vi "CAL_LOAD_R.vi"(9 "Control param In":T1={"L_velocity"=10000, "L_Power"=0.0, "R_velocity"=10000, "R_Power"=0.0, "T_param_L"={"Onset start"=0.0, "Onset end"=5.0, "Peak start"=10.0, "Release start"=60.0, "slang"=80.0, "Peak end"=58.0}, "T_param_R"={"Onset start"=0.0, "Onset end"=5.0, "Peak start"=10.0, "Release start"=60.0, "slang"=80.0, "Peak end"=58.0}, "Initialize?"=FALSE, "CAN read?"=FALSE, "Optimal count"=0}, 10 "Force":sgl[](array[numeric]), 11 "Param In":T2) -> (3 "Param Out":T2, 5 "Load_Peak":sgl, 7 "Load_Onset":sgl)   [LabVIEW 2019]
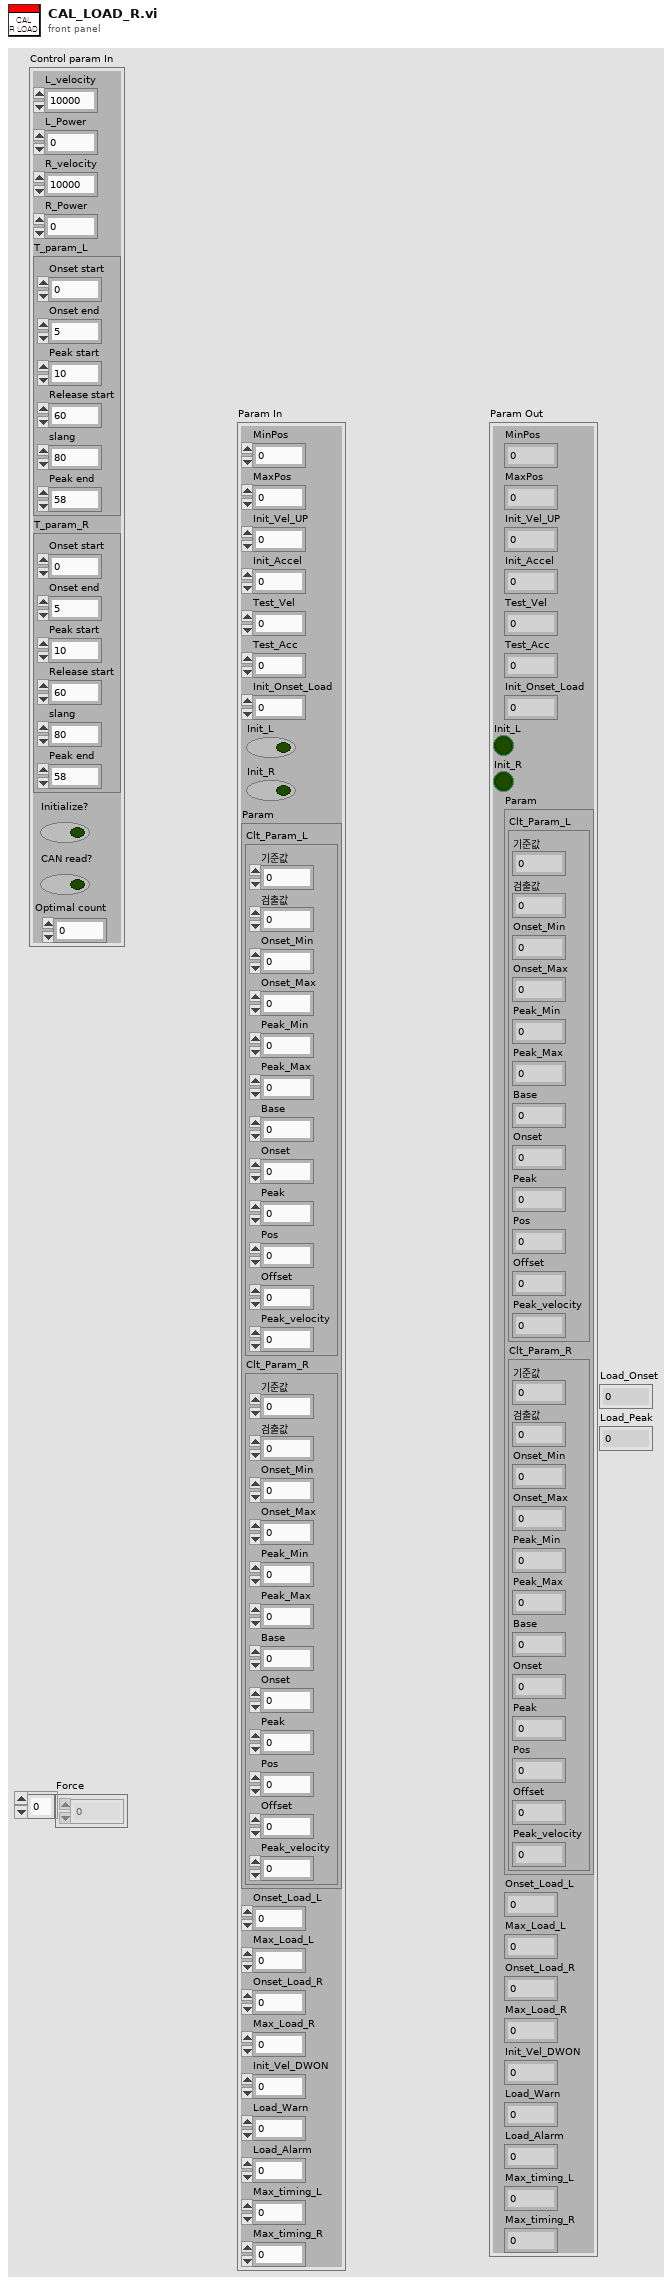
[diagram p1: front panel]
types:
  T1 = cluster{"L_velocity":u32, "L_Power":sgl, "R_velocity":u32, "R_Power":sgl, "T_param_L":cluster{"Onset start":sgl, "Onset end":sgl, "Peak start":sgl, "Release start":sgl, "slang":sgl, "Peak end":sgl}, "T_param_R":cluster{"Onset start":sgl, "Onset end":sgl, "Peak start":sgl, "Release start":sgl, "slang":sgl, "Peak end":sgl}, "Initialize?":bool, "CAN read?":bool, "Optimal count":i32}
  T2 = cluster{"MinPos":i32, "MaxPos":i32, "Init_Vel_UP":i32, "Init_Accel":u32, "Test_Vel":i32, "Test_Acc":u32, "Init_Onset_Load":sgl, "Init_L":bool, "Init_R":bool, "Param":cluster{"Clt_Param_L":cluster{"기준값":sgl, "검출값":sgl, "Onset_Min":sgl, "Onset_Max":sgl, "Peak_Min":sgl, "Peak_Max":sgl, "Base":i32, "Onset":i32, "Peak":i32, "Pos":i32, "Offset":sgl, "Peak_velocity":i32}, "Clt_Param_R":cluster{"기준값":sgl, "검출값":sgl, "Onset_Min":sgl, "Onset_Max":sgl, "Peak_Min":sgl, "Peak_Max":sgl, "Base":i32, "Onset":i32, "Peak":i32, "Pos":i32, "Offset":sgl, "Peak_velocity":i32}}, "Onset_Load_L":sgl, "Max_Load_L":sgl, "Onset_Load_R":sgl, "Max_Load_R":sgl, "Init_Vel_DWON":i32, "Load_Warn":sgl, "Load_Alarm":sgl, "Max_timing_L":sgl, "Max_timing_R":sgl}
  T3 = cluster{"Onset start":sgl, "Onset end":sgl, "Peak start":sgl, "Release start":sgl, "slang":sgl, "Peak end":sgl}
  T4 = cluster{"Onset start":i32, "Onset end":i32, "Peak start":i32, "Release start":i32, "slang":i32, "Peak end":i32}
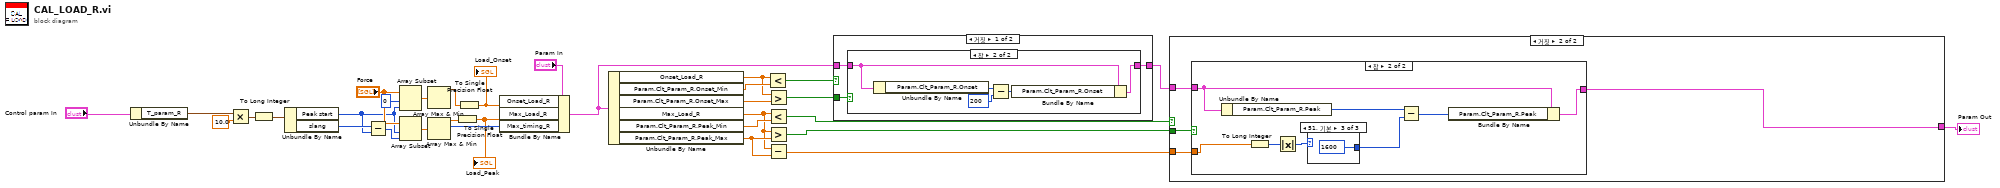
[diagram p0: block diagram]
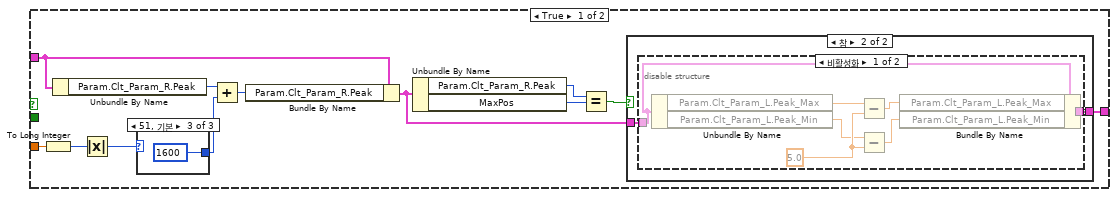
[diagram p2: hidden frame]
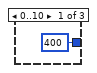
[diagram p5: hidden frame]
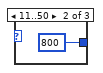
[diagram p6: hidden frame]
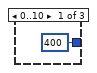
[diagram p8: hidden frame]
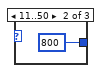
[diagram p9: hidden frame]
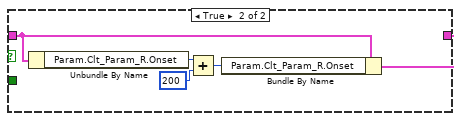
[diagram p11: hidden frame]
diagram:
  n1 = Unbundle By Name("Control param In") -> ("T_param_R"=w6:T3)
  n2 = Multiply(x=w6, y=sgl 10.0) -> (x*y=w22:T3)
  n3 = To Long Integer(number=w22) -> (32bit integer=w21:T4)
  n4 = Unbundle By Name(w21) -> ("Peak start"=w7:i32, "slang"=w14:i32)
  n5 = Subtract(x=w14, y=w7) -> (x-y=w8:i32)
  n6 = Array Subset(array="Force", index=0 ("인덱스"), length=w7) -> (w18:sgl[])
  n7 = Array Subset(array="Force", index=w7, length=w8) -> (w16:sgl[])
  n8 = Array Max & Min(array=w18) -> (max value=w10:sgl)  [unwired: 3 out]
  n9 = Array Max & Min(array=w16) -> (max value=w12:sgl, max index (indices)=w13:i32)  [unwired: 2 out]
  n10 = To Single Precision Float(number=w12) -> (single precision float=w11:sgl)
  "Load_Peak" <- w11
  n11 = To Single Precision Float(number=w10) -> (single precision float=w9:sgl)
  "Load_Onset" <- w9
  n12 = Bundle By Name(cluster="Param In", "Onset_Load_R"=w9, "Max_Load_R"=w11, "Max_timing_R"=w13) -> (w19:T2)
  n13 = Unbundle By Name(w19) -> ("Onset_Load_R"=w30:sgl, "Param.Clt_Param_R.Onset_Min"=w32:sgl, "Param.Clt_Param_R.Onset_Max"=w31:sgl, "Max_Load_R"=w2:sgl, "Param.Clt_Param_R.Peak_Min"=w29:sgl, "Param.Clt_Param_R.Peak_Max"=w3:sgl)
  n14 = Less?(x=w30, y=w32) -> (x < y?=w28:bool)
  n15 = Greater?(x=w30, y=w31) -> (0:w27:bool)
  n16 = Less?(x=w2, y=w29) -> (x < y?=w25:bool)
  n17 = Greater?(x=w2, y=w3) -> (0:w24:bool)
  n18 = Subtract(x=w2, y=w3) -> (x-y=w1:sgl)
  n19 = case shown="거짓" w28 {
    tunnel: w19 -> [w35 w43]
    tunnel: w27 -> [w33 _]
    tunnel: [w34 w42] -> w26
    frame False {
      n20 = case shown="참" w33 {
        tunnel: w35 -> [w36 w39]
        tunnel: [w36 w37] -> w34
        frame False {
        }
        frame True {
          n21 = Unbundle By Name(w39) -> ("Param.Clt_Param_R.Onset"=w41:i32)
          n22 = Subtract(x=w41, y=200) -> (x-y=w38:i32)
          n23 = Bundle By Name(cluster=w39, "Param.Clt_Param_R.Onset"=w38) -> (w37:T2)
        }
      }
    }
    frame True {
      n24 = Unbundle By Name(w43) -> ("Param.Clt_Param_R.Onset"=w46:i32)
      n25 = Add(x=w46, y=200) -> (x+y=w44:i32)
      n26 = Bundle By Name(cluster=w43, "Param.Clt_Param_R.Onset"=w44) -> (w42:T2)
    }
  }
  n27 = case shown="거짓" w25 {
    tunnel: w26 -> [w56 w76]
    tunnel: [w50 w75] -> w5
    tunnel: w24 -> [_ w74]
    tunnel: w1 -> [w47 w73]
    frame True {
      n28 = To Long Integer(number=w47) -> (32bit integer=w49:i32)
      n29 = Unbundle By Name(w56) -> ("Param.Clt_Param_R.Peak"=w58:i32)
      n30 = Absolute Value(x=w49) -> (abs(x)=w48:i32)
      n31 = case shown="51, 기본" w48 {
        tunnel: [400 ("y") 800 ("y") 1600 ("y")] -> w55
        frame 0..10 {
        }
        frame 11..50 {
        }
        frame 51, Default {
        }
      }
      n32 = Add(x=w58, y=w55) -> (x+y=w57:i32)
      n33 = Bundle By Name(cluster=w56, "Param.Clt_Param_R.Peak"=w57) -> (w51:T2)
      n34 = Unbundle By Name(w51) -> ("Param.Clt_Param_R.Peak"=w54:i32, "MaxPos"=w53:i32)
      n35 = Equal?(x=w54, y=w53) -> (x = y?=w52:bool)
      n36 = case shown="참" w52 {
        tunnel: w51 -> [w59 w61]
        tunnel: [w59 w60] -> w50
        frame False {
        }
        frame True {
          n37 = disable-structure shown="비활성화" {
            disable-tunnel: w61 -> [w63 w69]
            disable-tunnel: [w62 w69] -> w60
            frame Disabled {
              w68 = sgl 5.0
              n38 = Unbundle By Name(w63) -> ("Param.Clt_Param_L.Peak_Max"=w67:sgl, "Param.Clt_Param_L.Peak_Min"=w64:sgl)
              n39 = Subtract(x=w67, y=w68) -> (x-y=w66:sgl)
              n40 = Subtract(x=w64, y=w68) -> (x-y=w65:sgl)
              n41 = Bundle By Name(cluster=w63, "Param.Clt_Param_L.Peak_Max"=w66, "Param.Clt_Param_L.Peak_Min"=w65) -> (w62:T2)
            }
            frame Enabled {
            }
          }
        }
      }
    }
    frame False {
      n42 = case shown="참" w74 {
        tunnel: w76 -> [w77 w84]
        tunnel: [w77 w82] -> w75
        tunnel: w73 -> [_ w79]
        frame False {
        }
        frame True {
          n43 = Unbundle By Name(w84) -> ("Param.Clt_Param_R.Peak"=w85:i32)
          n44 = To Long Integer(number=w79) -> (32bit integer=w81:i32)
          n45 = Absolute Value(x=w81) -> (abs(x)=w80:i32)
          n46 = case shown="51, 기본" w80 {
            tunnel: [400 ("y") 800 ("y") 1600 ("y")] -> w78
            frame 0..10 {
            }
            frame 11..50 {
            }
            frame 51, Default {
            }
          }
          n47 = Subtract(x=w85, y=w78) -> (x-y=w83:i32)
          n48 = Bundle By Name(cluster=w84, "Param.Clt_Param_R.Peak"=w83) -> (w82:T2)
        }
      }
    }
  }
  "Param Out" <- w5
